vi "Main (not complete).vi"() -> ()   [LabVIEW 2012]
panel:
  out "Distance in cm (US FL)":i16
  out "Distance in cm (US FR)":i16
  out "Distance in cm (US BK)":i16
  in  "6DOF robot arm controls":T1={"Axis 1 \n(base)"=1250, "Axis 2"=1600, "Axis 3"=1000, "Axis 4"=1900, "Axis 5"=1300, "Axis 6 \n(claw)"=1550} {"Axis 1 \n(base)" scale=500.0..2000.0; "Axis 2" scale=500.0..2000.0; "Axis 3" scale=500.0..2000.0; "Axis 4" scale=500.0..2000.0; "Axis 5" scale=500.0..2000.0; "Axis 6 \n(claw)" scale=500.0..2000.0}
  out "Horizontal Graduated Bar":sgl(slide) scale=11.1..12.6
  out "NMEA sentences":string
  out "Latitude [deg]":string
  out "Longitude [deg]":string
  out "UTC Time":string
  out "Speed over ground [knots]":string
  out "Course over ground [degrees]":string
  out "Date [ddmmyy]":string
  out "Mode":string
  out "String 5":string
  out "String 4":string
  out "String 3":string
  out "String 2":string
  out "PIR (Living being detection)":bool
  in  "LED3":u8(slide) scale=0.0..100.0
  in  "LED2":u8(slide) scale=0.0..100.0
  in  "LED1":u8(slide) scale=0.0..100.0
  in  "LED0":u8(slide) scale=0.0..100.0
  out "Image":T2(plugin-control)
  in  "Capture":bool
  in  "Image Logging path":path
  out "Number of Frames":u32
  out "Frame Rate":dbl
  in  "Acquire?":bool
  in  "Up Button":bool
  in  "Right Button":bool caption="Next Button"
  in  "Left Button":bool
  in  "Down Button":bool
  in  "Stop Button":bool
  # "LED brightness controls\n (they can be used\n to attract attention)"
  # "Use the arrow keys to on your\nlaptop/desktop keyboard to control\nthe robot's movement"
  # "BMP180 Data"
  # "Ultrasound"
  # "Allow a few seconds after the button\nis pressed for the code to stop"
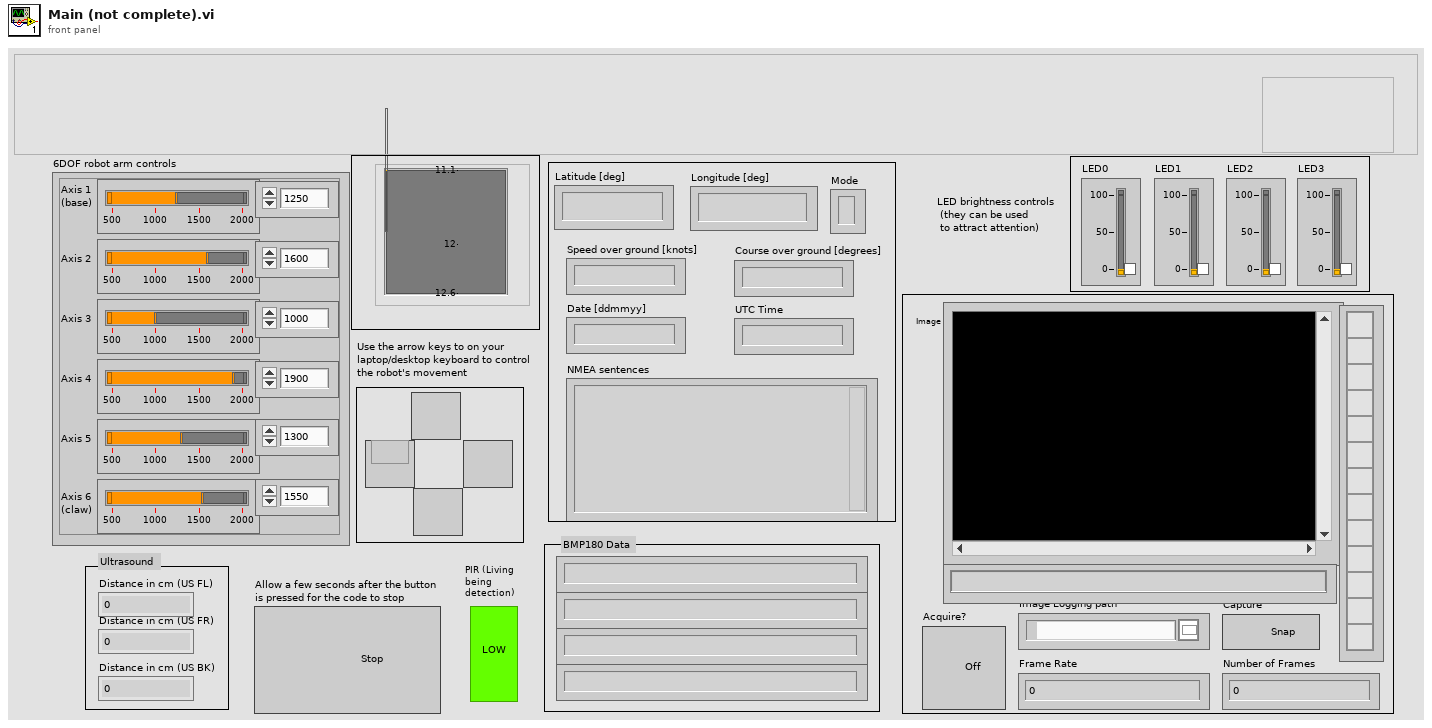
[diagram p1: front panel]
types:
  T1 = cluster{"Axis 1 \n(base)":i16, "Axis 2":i16, "Axis 3":i16, "Axis 4":i16, "Axis 5":i16, "Axis 6 \n(claw)":i16}
  T2 = typedef "IMAQ Image.ctl" = refnum<image>
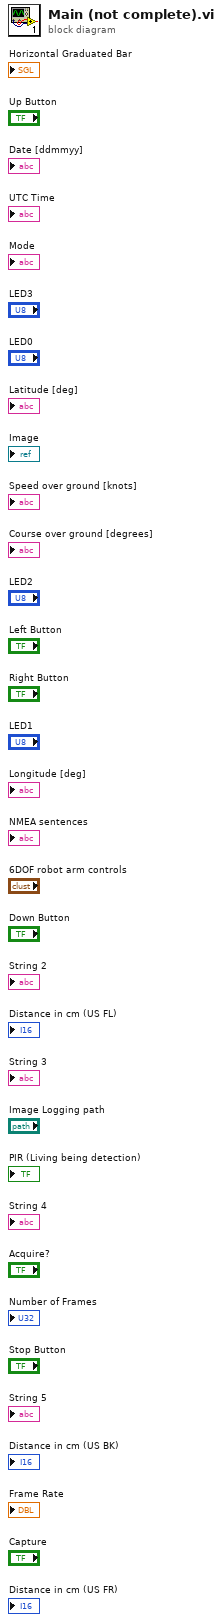
[diagram p0: block diagram]
diagram:
